vi "Camera.Piezo.vi"() -> ()   [LabVIEW 2015]
uses:
  Camera Properties.ctl
  CameraState.ctl
  CameraControlTypeDef.ctl
  Stack_State.ctl
  Stack Track.ctl
  <vilib>/vision/NI_Vision_Development_Module.lvlib
panel:
  in  "Tab Control":enum32{"Camera Settings", "Recording"}(tab)
  in  "Camera Mode":T1(ring)
  in  "Slit Width /px":dbl
  out "error IO":errorcluster
  in  "V Height":dbl=2048.0 min=4.0 max=2048.0 step=4.0
  in  "V Offset":dbl min=0.0 max=0.0 step=4.0
  in  "H Offset":dbl min=0.0 max=0.0 step=4.0
  in  "H Width":dbl min=4.0 max=2048.0 step=4.0
  in  "Exposure /ms":dbl min=0.0010036691729323308 max=10.000004210526315 step=1e-08
  in  "Trigger Source":dbl(ring)=2.0 items=["Internal"=1.0, "External"=2.0]
  in  "Readout Direction":dbl(ring)=2.0 items=["Forward"=1.0, "Backward"=2.0]
  in  "Scanning Mode":dbl(ring)=12.0 items=["Full Frame"=1.0, "Slit Scanning"=12.0]
  in  "Advanced DCAM Controls":i32(listbox) caption="Multicolumn Listbox"
  in  "Properties":T2=4211904 items=["SENSOR MODE"=4212128, "CCD MODE"=4212384, "READOUT MODE"=4211872, "ACTIVE VIEW INDEX"=4343136, "BITS PER CHANNEL"=4342976, "IMAGE PIXEL TYPE"=4343296, "BINNING"=4215968, "EXPOSURE TIME"=2049184, "CONTRAST GAIN"=3163312, "CONTRAST OFFSET"=3163328, "LIGHT MODE"=2114720, "SENSITIVITY"=2114992, "PHOTON IMAGING MODE"=2115200, "HIGH DYNAMIC RANGE MODE"=3163360, "WHITE BALANCE"=3163568, "TEMPERATURE"=2115232, "TEMPERATURE TARGET"=2115264, "SENSOR COOLER FAN"=2115296, "LINEBUNDLE HEIGHT"=4212192, "MECHANICAL SHUTTER"=2115488, "BACK FOCUS POSITION"=8422304, "TRIGGER CONNECTOR"=1066432, "TRIGGER SOURCE"=1066144, "OUTPUT TRIGGER SOURCE"=1852576, "TRIGGER GLOBAL EXPOSURE"=2049680, "FIRST TRIGGER BEHAVIOR"=2049696, "CHANNEL SYNC"=1852352, "READOUT DIRECTION"=4211904, "PRE HSYNC COUNT"=1852704, "INTERNAL LINE SPEED"=4191408, "INTERNAL LINE INVERVAL"=4191424]
  out "Image":T3(plugin-control)
  out "Histogram":T4(graph)
  in  "stop":bool
  in  "Calibration":bool
  in  "MultiD Scan":bool
  in  "Stage Controller":bool
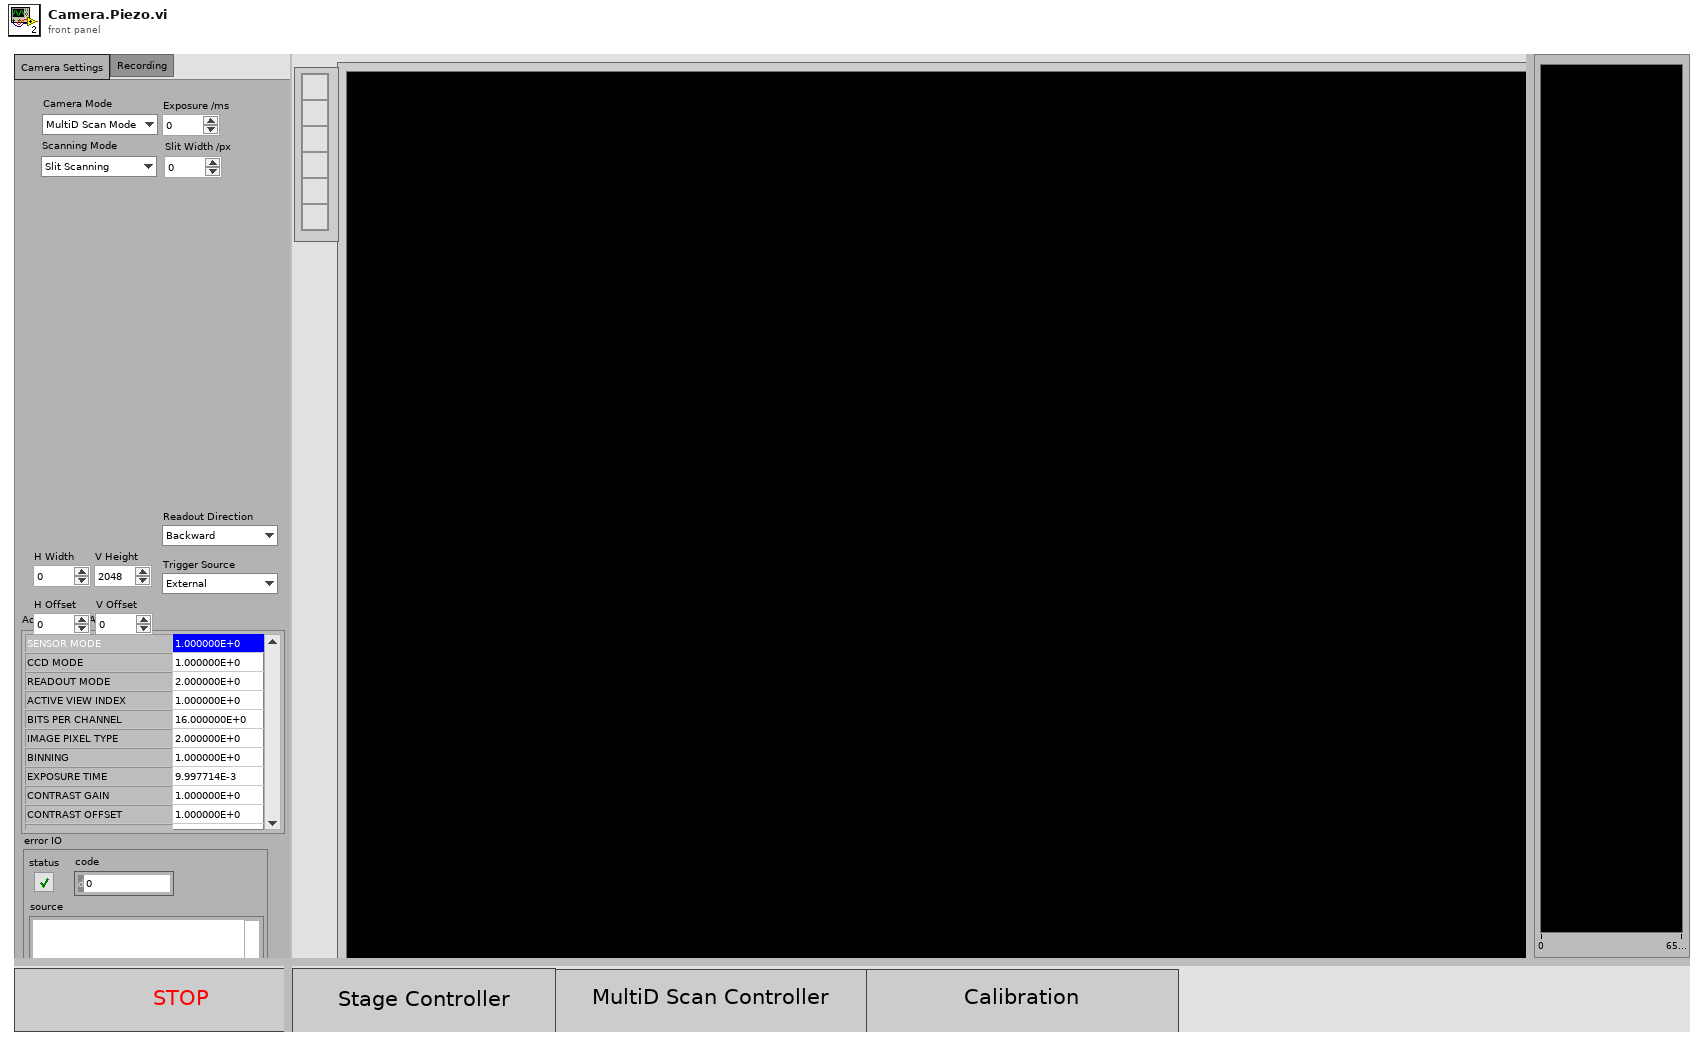
[diagram p1: front panel]
types:
  T1 = enum16{"MultiD Scan Mode", "2D Scan Mode", "Calibration Mode"}
  T2 = typedef "Camera Properties.ctl" = u32
  T3 = typedef "IMAQ Image.ctl" = refnum<image>
  T4 = cluster{"Starting Value":sgl, "Incremental Value":sgl, "Histogram":u32[]}
  T5 = typedef "CameraControlTypeDef.ctl" = enum16{"IntervalLineInt", "Ram Record", "HardDisk Record", "Disengage Update", "Update", "Idle", "ROI", "Binning", "Scan Mode", "Trigger Mode", "Readout Mode", "Readout Direction", "Preview", "ROIWindow", "Trigger Source"}
  T6 = cluster{"height":u32, "width":u32, "datatype":u32}
  T7 = typedef "Stack_State.ctl" = cluster{"State":T8, "Stack Number":i32, "Image":u16[][], "Stacks":i32}
  T8 = typedef "Stack Track.ctl" = enum16{"Idle", "Display", "Start Sequence", "Read Disk", "STOP", "Collecting", "End"}
  T9 = typedef "CameraState.ctl" = enum16{"init", "active", "deinit"}
  T10 = typedef "Image Type" = u32
  T11 = cluster{"Value":i32, "Minimum":i32, "Maximum":i32, "Increment":i32}
  T12 = cluster{"Minimum":i32, "Maximum":i32, "Increment":i32}
  T13 = cluster{"Enum":T5, dbl, "timeout in ms (-1)":u32}
  T14 = cluster{"State":T8, "Timeout":i32, "Data 16":u16[][], "Timeout":i32}
  T15 = cluster{"Enum":T5, "Trigger Source":dbl, "timeout in ms (-1)":i32}
  T16 = cluster{"Enum":T5, "Exposure /ms":dbl, "Parameter":u32}
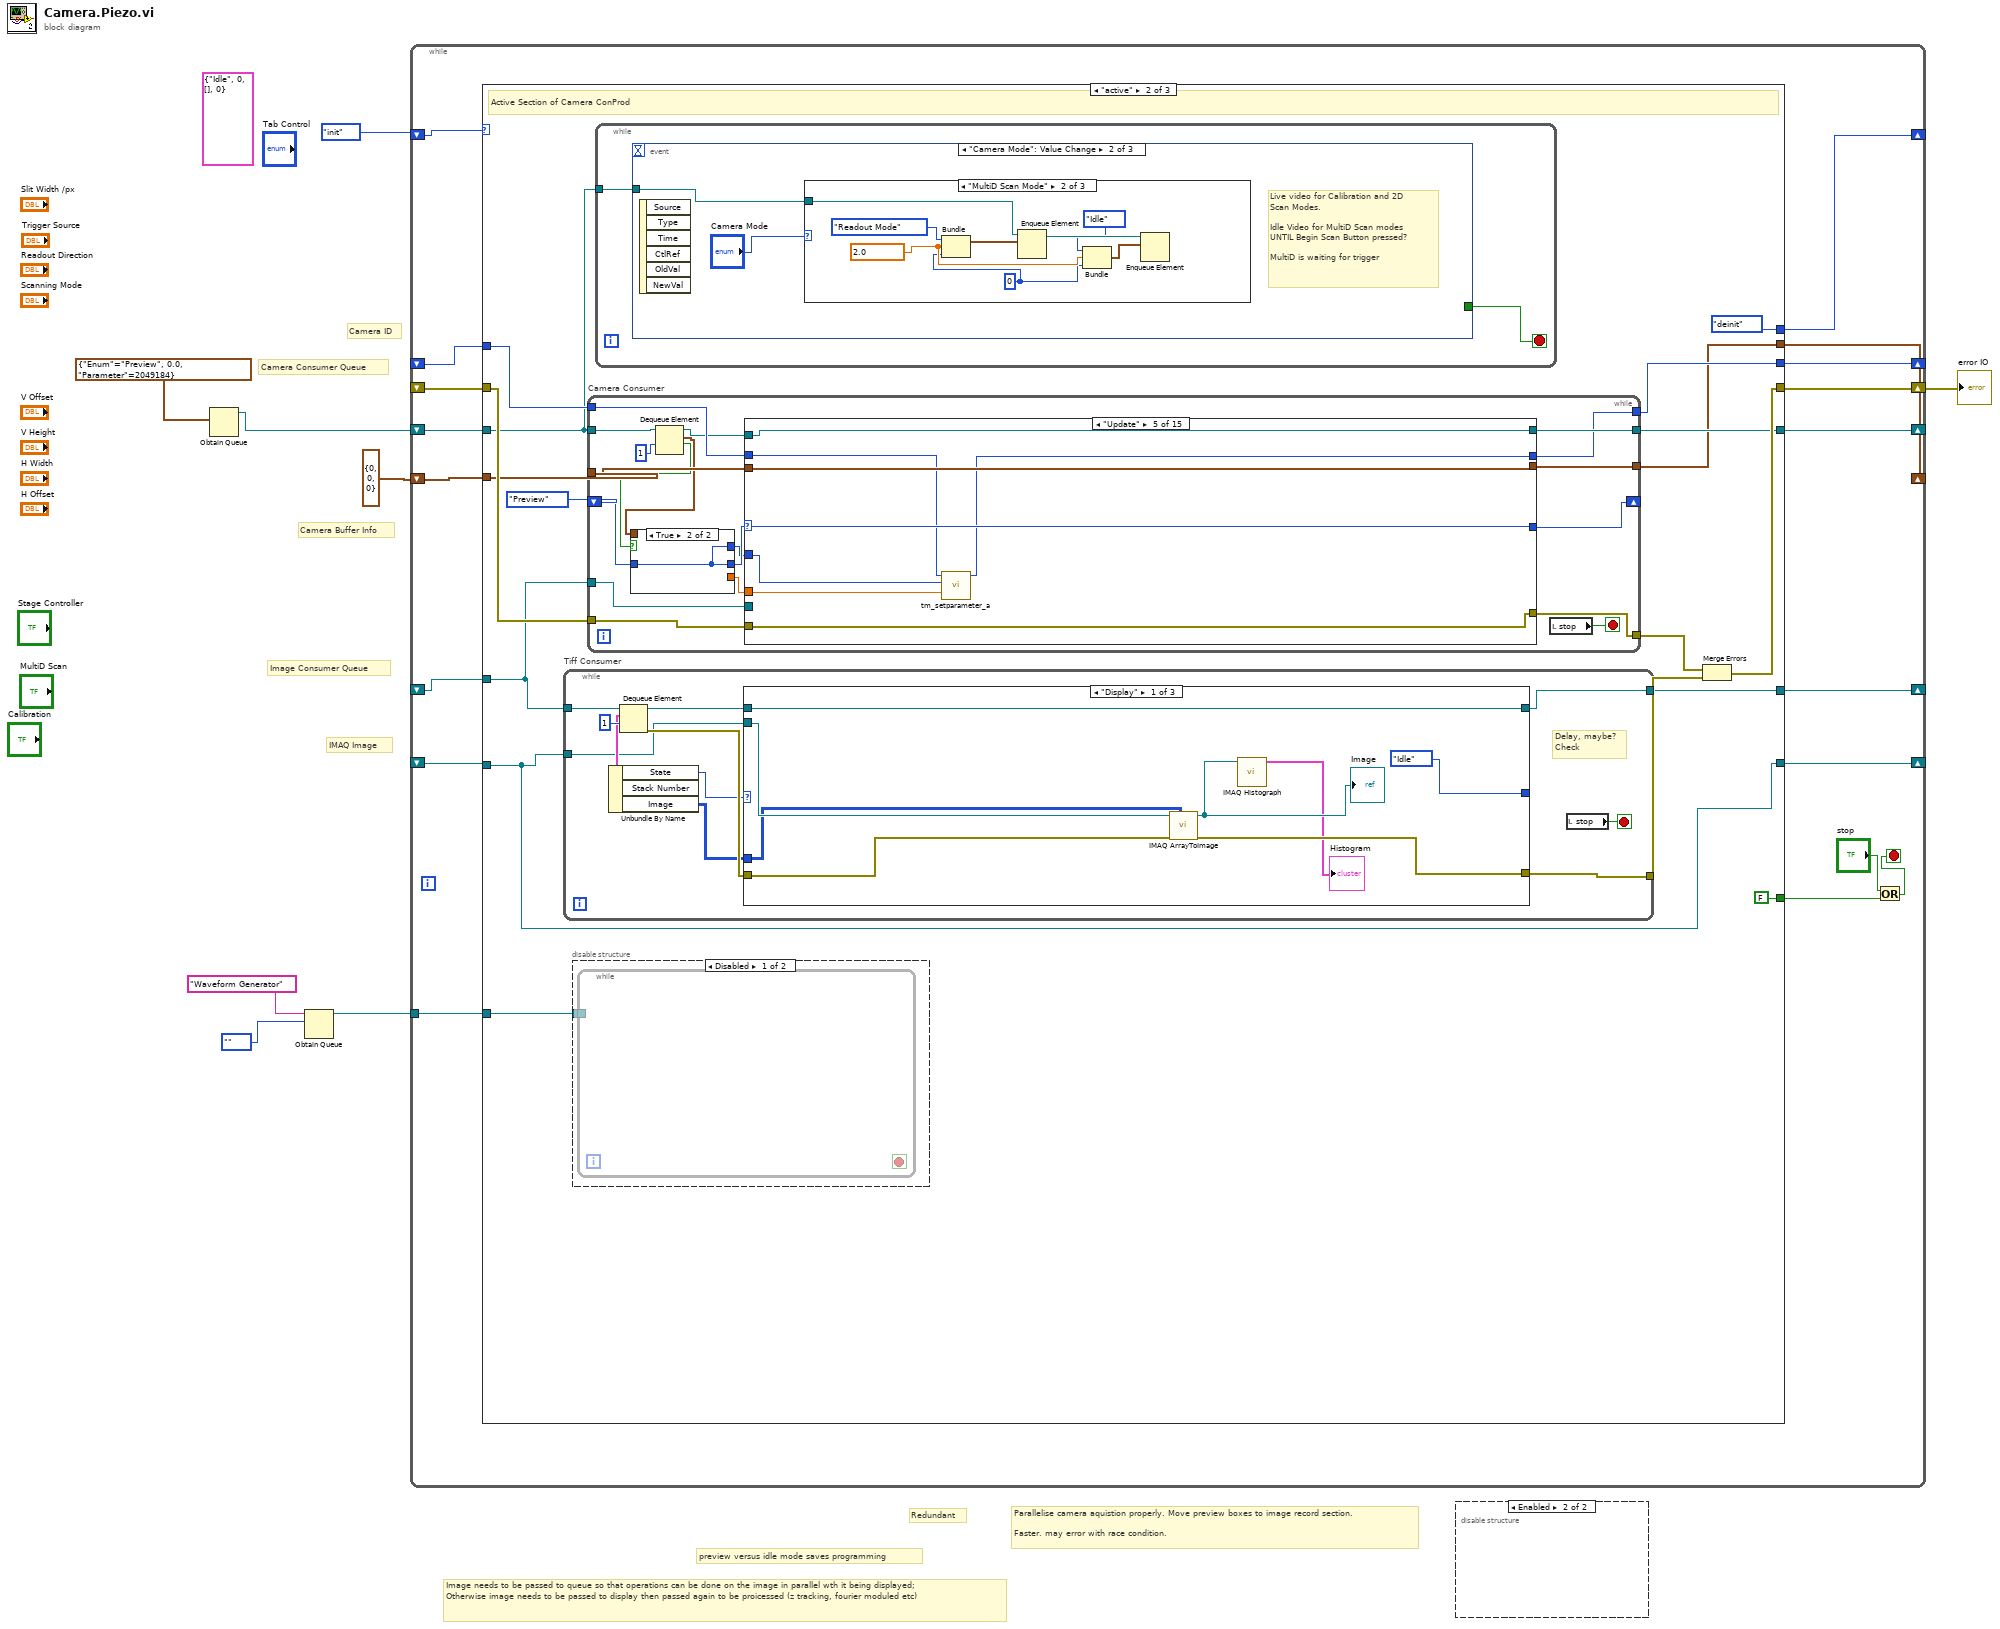
[diagram p0: block diagram]
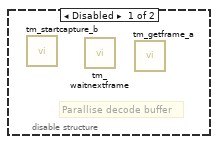
[diagram p2: hidden frame]
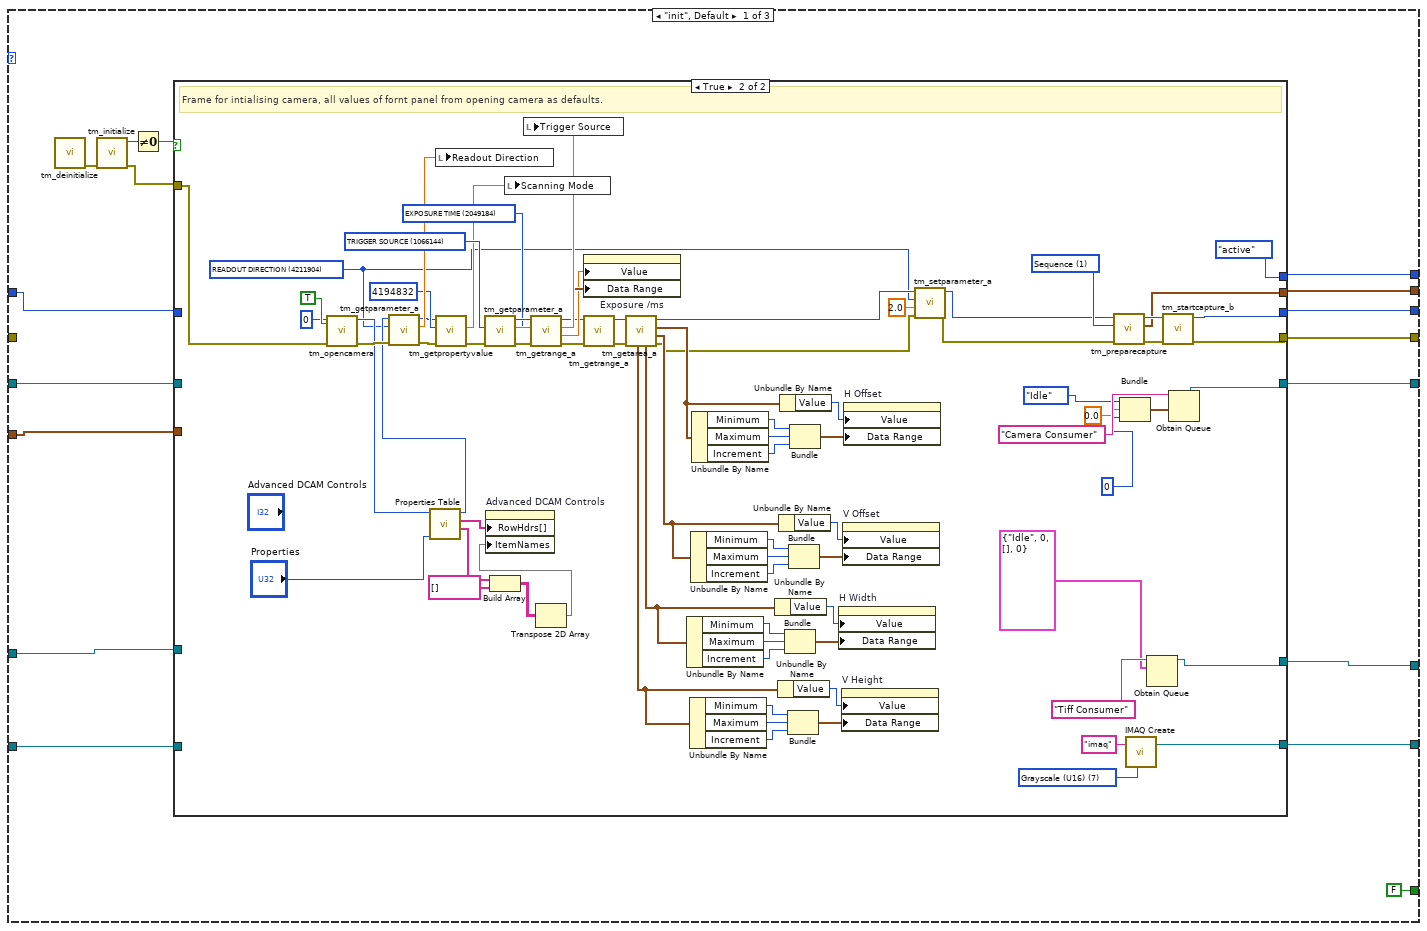
[diagram p3: hidden frame]
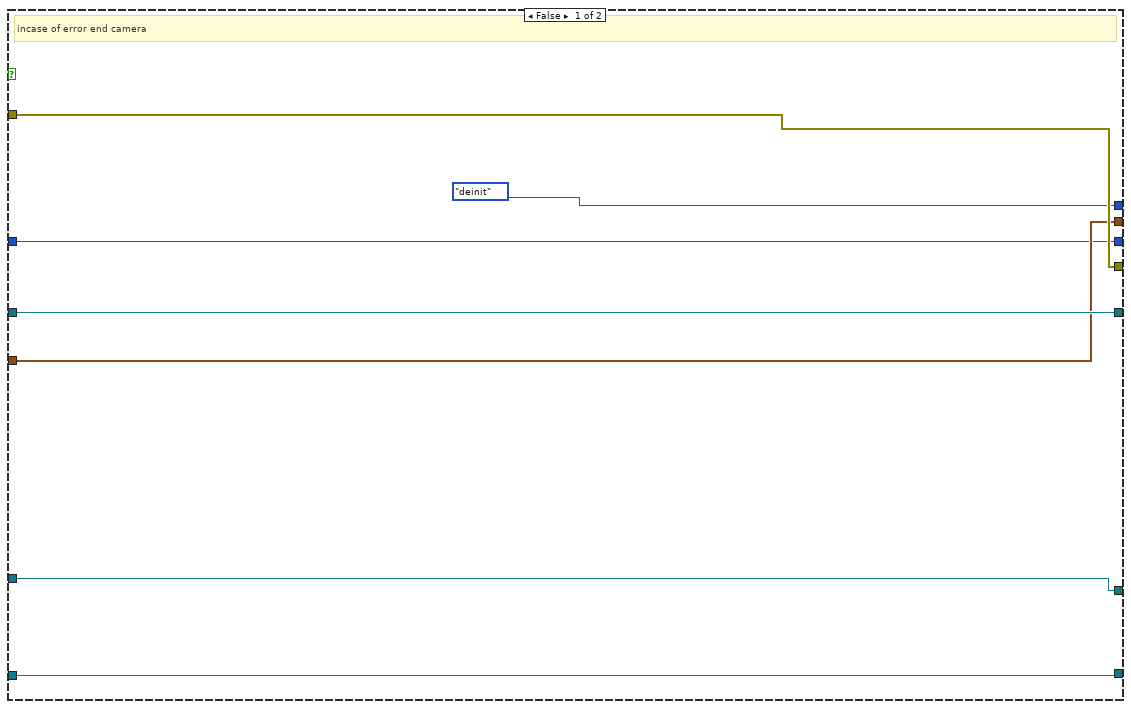
[diagram p4: hidden frame]
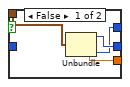
[diagram p8: hidden frame]
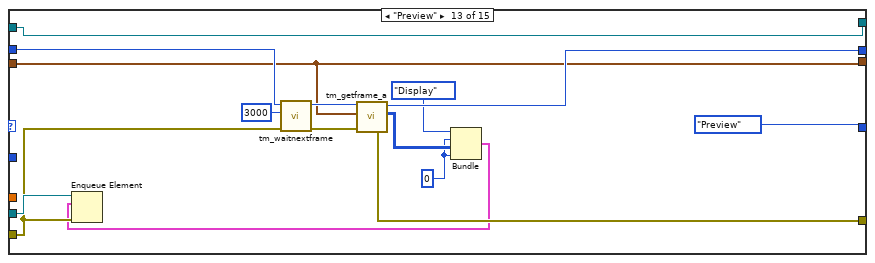
[diagram p20: hidden frame]
diagram:
  (unwired) T7 {"State"=enum."Idle", "Stack Number"=0, "Image"=[], "Stacks"=0} ("input cluster")
  # "IMAQ Image"
  # "Camera Buffer Info"
  # "Image needs to be passed to queue so that operations can be done on the image in parallel wth it being displayed;\nOtherwise image needs to be passed to display then passed again to be proicessed (z tracking, fourier moduled etc)"
  # "preview versus idle mode saves programming"
  # "Parallelise camera aquistion properly. Move preview boxes to image record section.\n\nFaster. may error with race condition."
  # "Redundant"
  # "Image Consumer Queue"
  # "Camera Consumer Queue"
  # "Camera ID"
  n1 = Obtain Queue(element data type=cluster{"Enum":T5, dbl, "Parameter":u32} {"Enum"=enum."Preview", 0.0, "Parameter"=2049184}) -> (queue out=w3:refnum<queue>)  [unwired: 4 in, 2 out]
  n2 = Obtain Queue(name (unnamed)="Waveform Generator", element data type=enum16{""}."") -> (queue out=w2:refnum<queue>)  [unwired: 3 in, 2 out]
  n3 = while {
    shift-right: [w26] -> _
    shift-left: CameraState."init" -> [w25]
    shift-right: [w24] -> _
    shift-left: _ -> [w23]
    shift-right: [w22] -> w7
    shift-left: _ -> [w21]
    shift-right: [w19] -> _
    shift-left: _ -> [w18]
    shift-right: [w20] -> _
    shift-left: w3 -> [w17]
    shift-right: [w13] -> _
    shift-left: T6 {"height"=0, "width"=0, "datatype"=0} ("Buffer Info") -> [w12]
    shift-right: [w11] -> _
    shift-left: _ -> [w10]
    tunnel: w2 -> [w9]
    stop <- w15 stop-if-true
    n4 = case shown="\"active\"" w25 {
      tunnel: [w39 CameraState."deinit" CameraState."init"] -> w26
      tunnel: [w38 w144 w324] -> w24
      tunnel: w23 -> [w29 w145 w324]
      tunnel: [w37 w143 w327] -> w22
      tunnel: w21 -> [_ w137 w328]
      tunnel: [w36 w140 w321] -> w20
      tunnel: [w35 w139 w322] -> w19
      tunnel: w18 -> [w33 w132 w322]
      tunnel: w17 -> [w34 w130 w321]
      tunnel: [FALSE ("stop") FALSE ("stop") TRUE ("stop")] -> w14
      tunnel: [w31 w135 w319] -> w13
      tunnel: w12 -> [w30 w134 w319]
      tunnel: w10 -> [w27 w131 w318]
      tunnel: [w28 w131 w318] -> w11
      tunnel: w9 -> [_ w129 _]
      frame "init", Default {
        n5 = call "tm_deinitialize.vi"() -> ("error out"=w43:errorcluster)  [unwired: 11 in]
        n6 = call "tm_initialize.vi"("error in (no error)"=w43) -> ("error out"=w40:errorcluster, "Number Of Cameras"=w42:u32)  [unwired: 7 in, 2 out]
        n7 = Not Equal To 0?(x=w42) -> (x != 0?=w41:bool)
        n8 = case shown="True" w41 {
          tunnel: w40 -> [w50 w122]
          tunnel: [CameraState."deinit" CameraState."active"] -> w39
          tunnel: [w50 w105] -> w37
          tunnel: [w45 w103] -> w38
          tunnel: [w48 w77] -> w36
          tunnel: [w47 w75] -> w35
          tunnel: w34 -> [w48 _]
          tunnel: w33 -> [w47 _]
          tunnel: [w46 w65] -> w31
          tunnel: w30 -> [w46 _]
          tunnel: w29 -> [w45 _]
          tunnel: [w44 w62] -> w28
          tunnel: w27 -> [w44 _]
          frame False {
            # "incase of error end camera"
          }
          frame True {
            w64 = T10 7 items=["Grayscale (U8)", "Grayscale (I16)", "Grayscale (SGL)", "Complex (CSG)", "RGB (U32)", "HSL (U32)", "RGB (U64)", "Grayscale (U16)"] ("Image Type")
            w107 = 1 items=["Snap", "Sequence"] ("Capture mode")
            w119 = u32 2049184 items=["SENSOR MODE"=4212128, "CCD MODE"=4212384, "READOUT MODE"=4211872, "ACTIVE VIEW INDEX"=4343136, "BITS PER CHANNEL"=4342976, "IMAGE PIXEL TYPE"=4343296, "BINNING"=4215968, "EXPOSURE TIME"=2049184, "CONTRAST GAIN"=3163312, "CONTRAST OFFSET"=3163328, "LIGHT MODE"=2114720, "SENSITIVITY"=2114992, "PHOTON IMAGING MODE"=2115200, "HIGH DYNAMIC RANGE MODE"=3163360, "WHITE BALANCE"=3163568, "TEMPERATURE"=2115232, "TEMPERATURE TARGET"=2115264, "SENSOR COOLER FAN"=2115296, "LINEBUNDLE HEIGHT"=4212192, "MECHANICAL SHUTTER"=2115488, "BACK FOCUS POSITION"=8422304, "TRIGGER CONNECTOR"=1066432, "TRIGGER SOURCE"=1066144, "OUTPUT TRIGGER SOURCE"=1852576, "TRIGGER GLOBAL EXPOSURE"=2049680, "FIRST TRIGGER BEHAVIOR"=2049696, "CHANNEL SYNC"=1852352, "READOUT DIRECTION"=4211904, "PRE HSYNC COUNT"=1852704, "INTERNAL LINE SPEED"=4191408, "INTERNAL LINE INVERVAL"=4191424] ("Parameter")
            w57 = T2 4211904 items=["SENSOR MODE"=4212128, "CCD MODE"=4212384, "READOUT MODE"=4211872, "ACTIVE VIEW INDEX"=4343136, "BITS PER CHANNEL"=4342976, "IMAGE PIXEL TYPE"=4343296, "BINNING"=4215968, "EXPOSURE TIME"=2049184, "CONTRAST GAIN"=3163312, "CONTRAST OFFSET"=3163328, "LIGHT MODE"=2114720, "SENSITIVITY"=2114992, "PHOTON IMAGING MODE"=2115200, "HIGH DYNAMIC RANGE MODE"=3163360, "WHITE BALANCE"=3163568, "TEMPERATURE"=2115232, "TEMPERATURE TARGET"=2115264, "SENSOR COOLER FAN"=2115296, "LINEBUNDLE HEIGHT"=4212192, "MECHANICAL SHUTTER"=2115488, "BACK FOCUS POSITION"=8422304, "TRIGGER CONNECTOR"=1066432, "TRIGGER SOURCE"=1066144, "OUTPUT TRIGGER SOURCE"=1852576, "TRIGGER GLOBAL EXPOSURE"=2049680, "FIRST TRIGGER BEHAVIOR"=2049696, "CHANNEL SYNC"=1852352, "READOUT DIRECTION"=4211904, "PRE HSYNC COUNT"=1852704, "INTERNAL LINE SPEED"=4191408, "INTERNAL LINE INVERVAL"=4191424] ("Parameter")
            w125 = u32 1066144 items=["SENSOR MODE"=4212128, "CCD MODE"=4212384, "READOUT MODE"=4211872, "ACTIVE VIEW INDEX"=4343136, "BITS PER CHANNEL"=4342976, "IMAGE PIXEL TYPE"=4343296, "BINNING"=4215968, "EXPOSURE TIME"=2049184, "CONTRAST GAIN"=3163312, "CONTRAST OFFSET"=3163328, "LIGHT MODE"=2114720, "SENSITIVITY"=2114992, "PHOTON IMAGING MODE"=2115200, "HIGH DYNAMIC RANGE MODE"=3163360, "WHITE BALANCE"=3163568, "TEMPERATURE"=2115232, "TEMPERATURE TARGET"=2115264, "SENSOR COOLER FAN"=2115296, "LINEBUNDLE HEIGHT"=4212192, "MECHANICAL SHUTTER"=2115488, "BACK FOCUS POSITION"=8422304, "TRIGGER CONNECTOR"=1066432, "TRIGGER SOURCE"=1066144, "OUTPUT TRIGGER SOURCE"=1852576, "TRIGGER GLOBAL EXPOSURE"=2049680, "FIRST TRIGGER BEHAVIOR"=2049696, "CHANNEL SYNC"=1852352, "READOUT DIRECTION"=4211904, "PRE HSYNC COUNT"=1852704, "INTERNAL LINE SPEED"=4191408, "INTERNAL LINE INVERVAL"=4191424] ("Parameter")
            # "Frame for intialising camera, all values of fornt panel from opening camera as defaults."
            n9 = call "tm_opencamera.vi"("Force Open"=TRUE, "error in (no error)"=w122, "Camera Index"=u32 0) -> ("error out"=w126:errorcluster, "Handle out"=w73:u32)  [unwired: 6 in, 1 out]
            n10 = call "Properties Table.vi"("Properties"="Properties", "Handle In"=w73) -> ("Value Stirngs Out"=w70:string[], "Row Headers"=w71:string[], "Handle Out"=w72:u32)  [unwired: 3 in, 1 out]
            n11 = call "tm_getparameter_a.vi"("error in (no error)"=w126, "Parameter"=w57, "Handle in"=w72) -> ("error out"=w108:errorcluster, "Value out"=w123:dbl, "Handle out"=w111:u32)  [unwired: 6 in]
            n12 = local write "Readout Direction"(w123) -> ()
            n13 = call "tm_getpropertyvalue.vi"("error in (no error)"=w108, "Property ID"=u32 4194832, "Handle in"=w111) -> ("error out"=w109:errorcluster, "Value in"=w110:sgl)  [unwired: 6 in, 1 out]
            n14 = call "tm_getparameter_a.vi"("error in (no error)"=w109, "Parameter"=w125) -> ("error out"=w120:errorcluster, "Value out"=w124:dbl, "Handle out"=w121:u32)  [unwired: 7 in]
            n15 = Build Array(w70, string[] [] ("element")) -> (w68:string[][])
            n16 = local write "Scanning Mode"(w110) -> ()
            n17 = local write "Trigger Source"(w124) -> ()
            n18 = call "tm_getrange_a.vi"("error in (no error)"=w120, "Parameter"=w119, "Handle in"=w121) -> ("error out"=w115:errorcluster, "default"=w117:dbl, "Range"=w118:cluster{"min":dbl, "max":dbl, "step":dbl}, "Handle out"=w116:u32)  [unwired: 2 in, 3 out]
            n19 = Transpose 2D Array(2D array=w68) -> (transposed array=w67:string[][])
            n20 = property on="Advanced DCAM Controls" class="MCListbox (strict)"("RowHdrs[]"=w71, "ItemNames"=w67) -> ()  [unwired: 2 in, 2 out]
            n21 = property on="Exposure /ms" class="DigNum (strict)"("Value"=w117, "Data Range"=w118) -> ()  [unwired: 2 in, 2 out]
            n22 = call "tm_getrange_a.vi"("error in (no error)"=w115, "Handle in"=w116) -> ("error out"=w114:errorcluster, "Handle out"=w113:u32)  [unwired: 3 in, 5 out]
            n23 = call "tm_getarea_a.vi"("error in (no error)"=w114, "Handle in"=w113) -> ("error out"=w59:errorcluster, "V Offset"=w79:T11, "H Offset"=w102:T11, "Handle out"=w61:u32, "H Width"=w80:T11, "V Width"=w81:T11)  [unwired: 4 in]
            n24 = Unbundle By Name(w80) -> ("Minimum"=w91:i32, "Maximum"=w90:i32, "Increment"=w89:i32)
            n25 = Unbundle By Name(w81) -> ("Minimum"=w82:i32, "Maximum"=w83:i32, "Increment"=w84:i32)
            n26 = Unbundle By Name(w79) -> ("Minimum"=w92:i32, "Maximum"=w93:i32, "Increment"=w94:i32)
            n27 = Unbundle By Name(w102) -> ("Minimum"=w101:i32, "Maximum"=w100:i32, "Increment"=w99:i32)
            n28 = Unbundle By Name(w80) -> ("Value"=w87:i32)
            n29 = Unbundle By Name(w81) -> ("Value"=w86:i32)
            n30 = Unbundle By Name(w79) -> ("Value"=w96:i32)
            n31 = Unbundle By Name(w102) -> ("Value"=w97:i32)
            n32 = Bundle("Minimum"=w91, "Maximum"=w90, "Increment"=w89) -> (w88:T12)  [unwired: 1 in]
            n33 = Bundle("Minimum"=w82, "Maximum"=w83, "Increment"=w84) -> (w85:T12)  [unwired: 1 in]
            n34 = Bundle("Minimum"=w92, "Maximum"=w93, "Increment"=w94) -> (w95:T12)  [unwired: 1 in]
            n35 = Bundle("Minimum"=w101, "Maximum"=w100, "Increment"=w99) -> (w98:T12)  [unwired: 1 in]
            n36 = property on="H Width" class="DigNum (strict)"("Value"=w87, "Data Range"=w88) -> ()  [unwired: 2 in, 2 out]
            n37 = property on="V Height" class="DigNum (strict)"("Value"=w86, "Data Range"=w85) -> ()  [unwired: 2 in, 2 out]
            n38 = property on="V Offset" class="DigNum (strict)"("Value"=w96, "Data Range"=w95) -> ()  [unwired: 2 in, 2 out]
            n39 = property on="H Offset" class="DigNum (strict)"("Value"=w97, "Data Range"=w98) -> ()  [unwired: 2 in, 2 out]
            n40 = call "tm_setparameter_a.vi"("error in (no error)"=w59, "Value in"=2.0, "Parameter"=w57, "Handle in"=w61) -> ("error out"=w58:errorcluster, "Handle out"=w60:u32)  [unwired: 6 in]
            n41 = call "tm_preparecapture.vi"("error in (no error)"=w58, "Capture mode"=w107, "Handle in"=w60) -> ("error out"=w106:errorcluster, "Buffer Info"=w65:T6, "Handle out"=w104:u32)  [unwired: 5 in, 1 out]
            n42 = Bundle("Enum"=CameraControlTypeDef."Idle", 0.0, "timeout in ms (-1)"=u32 0) -> (w53:T13)  [unwired: 1 in]
            n43 = call "IMAQ Create"("Image Name"="imaq", "Image Type"=w64) -> ("New Image"=w62:T3)  [unwired: 3 in, 1 out]
            n44 = Obtain Queue(name (unnamed)="Tiff Consumer", element data type=T7 {"State"=enum."Idle", "Stack Number"=0, "Image"=[], "Stacks"=0} ("input cluster")) -> (queue out=w75:refnum<queue>)  [unwired: 3 in, 2 out]
            n45 = call "tm_startcapture_b.vi"("error in (no error)"=w106, "Handle in"=w104) -> ("error out"=w105:errorcluster, "Handle out"=w103:u32)  [unwired: 8 in]
            n46 = Obtain Queue(name (unnamed)="Camera Consumer", element data type=w53) -> (queue out=w77:refnum<queue>)  [unwired: 3 in, 2 out]
          }
        }
      }
      frame "active" {
        # "Active Section of Camera ConProd"
        n47 = while "Tiff Consumer" {
          tunnel: [w150] -> w142
          tunnel: [w153] -> w139
          tunnel: w132 -> [w155]
          tunnel: w131 -> [w147]
          stop <- w157 stop-if-true
          # "Delay, maybe?\nCheck"
          n48 = Dequeue Element(queue=w155, timeout in ms (-1)=1) -> (queue out=w152:refnum<queue>, element=w154:T7, error out=w151:errorcluster)  [unwired: 1 in, 1 out]
          n49 = Unbundle By Name(w154) -> ("State"=w148:T8, "Image"=w149:u16[][])  [unwired: 1 out]
          n50 = case shown="\"Display\"" w148 {
            selector: w148 -> [_ w168 w169]
            tunnel: [w165 w167 w170] -> w153
            tunnel: w152 -> [w165 w167 w170]
            tunnel: [Stack_Track."Idle" ("State") w168 w169] -> _
            tunnel: w149 -> [w160 _ _]
            tunnel: w147 -> [w164 _ _]
            tunnel: w151 -> [w163 w166 w171]
            tunnel: [w162 w166 w171] -> w150
            frame "Display" {
              n51 = call "IMAQ ArrayToImage"("Image Pixels (U16)"=w160, "error in (no error)"=w163, "Image"=w164) -> ("error out"=w162:errorcluster, "Image Out"=w159:T3)  [unwired: 7 in]
              "Image" <- w159
              n52 = call "IMAQ Histograph"("Image"=w159) -> ("Histogram Graph"=→"Histogram":T4)  [unwired: 7 in, 3 out]
            }
            frame "Idle", Default {
            }
            frame "Start Sequence" {
            }
          }
          n53 = local read "stop"() -> (w157:bool)
        }
        n54 = disable-structure shown="Disabled" {
          disable-tunnel: w129 -> [w146 _]
          frame Disabled {
            n55 = while {
              tunnel: w146 -> [_]
              stop <- _ stop-if-true
            }
          }
          frame Enabled {
          }
        }
        n56 = while "Camera Consumer" {
          tunnel: w137 -> [w188]
          tunnel: w145 -> [w185]
          tunnel: [w184] -> w144
          tunnel: [w187] -> w141
          tunnel: w130 -> [w180]
          tunnel: [w189] -> w140
          shift-right: [w186] -> _
          shift-left: CameraControlTypeDef."Preview" ("Enum") -> [w176]
          tunnel: [w183] -> w135
          tunnel: w134 -> [w182]
          tunnel: w132 -> [w175]
          stop <- w190 stop-if-true
          n57 = Dequeue Element(queue=w180, timeout in ms (-1)=1) -> (queue out=w179:refnum<queue>, element=w174:cluster{"Enum":T5, dbl, "Parameter":u32}, timed out?=w178:bool)  [unwired: 1 in, 1 out]
          n58 = case shown="True" w178 {
            tunnel: [w193 w195] -> w177
            tunnel: w176 -> [_ w195]
            tunnel: w174 -> [w194 _]
            tunnel: [w192 _] -> w173
            tunnel: [w191 w195] -> w172
            frame False {
              n59 = Unbundle(w194) -> ("Enum"=w193:T5, w192:dbl, "Parameter"=w191:u32)
            }
            frame True {
            }
          }
          n60 = case shown="\"Update\"" w177 {
            selector: w177 -> [w199 w204 w209 w214 w222 w227 w232 w237 w242 w247 w252 w257 _ w276 _]
            tunnel: w179 -> [w198 w205 w210 w215 w223 w228 w233 w238 w243 w248 w253 w258 w273 w278 w283]
            tunnel: [w198 w205 w210 w215 w223 w228 w233 w238 w243 w248 w253 w258 w273 w278 w283] -> w189
            tunnel: w188 -> [w200 w203 w208 w213 w221 w226 w231 w236 w241 w246 w251 w256 w263 w275 w281]
            tunnel: [w200 w203 w208 w213 w221 w226 w231 w236 w241 w246 w251 w256 w267 w275 w281] -> w187
            tunnel: [w199 w204 w209 w214 w222 w227 w232 w237 w242 w247 w252 w257 CameraControlTypeDef."Preview" ("Enum") w276 CameraControlTypeDef."Preview" ("Enum")] -> w186
            tunnel: w185 -> [w197 w202 w207 w212 w219 w225 w230 w235 w240 w245 w250 w255 w271 w277 w282]
            tunnel: [w197 w202 w207 w212 w218 w225 w230 w235 w240 w245 w250 w255 w269 w277 w282] -> w184
            tunnel: [w196 w201 w206 w211 w220 w224 w229 w234 w239 w244 w249 w254 w265 w274 w280] -> w183
            tunnel: w182 -> [w196 w201 w206 w211 w220 w224 w229 w234 w239 w244 w249 w254 w265 w274 w280]
            tunnel: w175 -> [_ _ _ _ _ _ _ _ _ _ _ _ w264 _ _]
            tunnel: w173 -> [_ _ _ _ w216 _ _ _ _ _ _ _ _ _ _]
            tunnel: w172 -> [_ _ _ _ w217 _ _ _ _ _ _ _ _ _ _]
            frame "IntervalLineInt" {
            }
            frame "Ram Record" {
            }
            frame "HardDisk Record" {
            }
            frame "Disengage Update" {
            }
            frame "Update" {
              n61 = call "tm_setparameter_a.vi"("Value in"=w216, "Parameter"=w217, "Handle in"=w219) -> ("Handle out"=w218:u32)  [unwired: 7 in, 1 out]
            }
            frame "Idle", Default {
            }
            frame "ROI" {
            }
            frame "Binning" {
            }
            frame "Scan Mode" {
            }
            frame "Trigger Mode" {
            }
            frame "Readout Mode" {
            }
            frame "Readout Direction" {
            }
            frame "Preview" {
              w260 = 0 ("Timeout")
              n62 = call "tm_waitnextframe.vi"("error in (no error)"=w263, "Timeout"=3000, "Handle in"=w271) -> ("error out"=w268:errorcluster, "Handle out"=w270:u32)  [unwired: 5 in, 2 out]
              n63 = call "tm_getframe_a.vi"("error in (no error)"=w268, "Buffer Info"=w265, "Handle in"=w270) -> ("error out"=w267:errorcluster, "Data 16"=w261:u16[][], "Handle out"=w269:u32)  [unwired: 4 in, 2 out]
              n64 = Bundle("State"=Stack_Track."Display", "Timeout"=w260, "Data 16"=w261, "Timeout"=w260) -> (w259:T14)  [unwired: 1 in]
              n65 = Enqueue Element(queue=w264, element=w259, error in (no error)=w263) -> ()  [unwired: 1 in, 3 out]
            }
            frame "ROIWindow" {
            }
            frame "Trigger Source" {
              n66 = call "tm_unpreparecapture.vi"() -> ()  [unwired: 10 in, 2 out]
              n67 = call "tm_setparameter_a.vi"() -> ()  [unwired: 10 in, 2 out]
              n68 = call "tm_preparecapture.vi"() -> ()  [unwired: 8 in, 4 out]
            }
          }
          n69 = local read "stop"() -> (w190:bool)
        }
        n70 = while {
          tunnel: w130 -> [w284]
          stop <- w285 stop-if-true
          n71 = event shown="[1] \"Camera Mode\": Value Change" {
            selector: _ -> [_ _ _]
            dyn-events: _ -> [_ _ _]
            timeout: _ -> [_ _ _]
            tunnel: [w286 _ _] -> w285
            tunnel: w284 -> [_ w287 w315]
            event "stop": Value Change {
              n72 = event-data() -> ()  [unwired: 1 in, 6 out]
              n73 = local read "stop"() -> (w286:bool)
            }
            event "Camera Mode": Value Change {
              # "Live video for Calibration and 2D\nScan Modes.\n\nIdle Video for MultiD Scan modes\nUNTIL Begin Scan Button pressed?\n\nMultiD is waiting for trigger"
              n74 = event-data() -> ()  [unwired: 1 in, 6 out]
              n75 = case shown="\"MultiD Scan Mode\"" "Camera Mode" {
                tunnel: w287 -> [w295 w303 w311]
                frame "Calibration Mode" {
                  w289 = 0 ("timeout in ms (-1)")
                  w290 = 1.0 items=["Internal"=1.0, "External"=2.0] ("Trigger Source")
                  n76 = Bundle("Enum"=CameraControlTypeDef."Readout Mode", "Trigger Source"=w290, "timeout in ms (-1)"=w289) -> (w294:T15)  [unwired: 1 in]
                  n77 = Enqueue Element(queue=w295, element=w294) -> (queue out=w292:refnum<queue>)  [unwired: 2 in, 2 out]
                  n78 = Bundle("Enum"=CameraControlTypeDef."Preview", "Trigger Source"=w290, "timeout in ms (-1)"=w289) -> (w293:T15)  [unwired: 1 in]
                  n79 = Enqueue Element(queue=w292, element=w293) -> ()  [unwired: 2 in, 3 out]
                }
                frame "MultiD Scan Mode" {
                  w297 = 0 ("timeout in ms (-1)")
                  w298 = 2.0 items=["Internal"=1.0, "External"=2.0] ("Trigger Source")
                  n80 = Bundle("Enum"=CameraControlTypeDef."Readout Mode", "Trigger Source"=w298, "timeout in ms (-1)"=w297) -> (w302:T15)  [unwired: 1 in]
                  n81 = Enqueue Element(queue=w303, element=w302) -> (queue out=w301:refnum<queue>)  [unwired: 2 in, 2 out]
                  n82 = Bundle("Enum"=CameraControlTypeDef."Idle", "Trigger Source"=w298, "timeout in ms (-1)"=w297) -> (w300:T15)  [unwired: 1 in]
                  n83 = Enqueue Element(queue=w301, element=w300) -> ()  [unwired: 2 in, 3 out]
                }
                frame "2D Scan Mode" {
                  w305 = 0 ("timeout in ms (-1)")
                  w306 = 2.0 items=["Internal"=1.0, "External"=2.0] ("Trigger Source")
                  n84 = Bundle("Enum"=CameraControlTypeDef."Readout Mode", "Trigger Source"=w306, "timeout in ms (-1)"=w305) -> (w310:T15)  [unwired: 1 in]
                  n85 = Enqueue Element(queue=w311, element=w310) -> (queue out=w307:refnum<queue>)  [unwired: 2 in, 2 out]
                  n86 = Bundle("Enum"=CameraControlTypeDef."Preview", "Trigger Source"=w306, "timeout in ms (-1)"=w305) -> (w309:T15)  [unwired: 1 in]
                  n87 = Enqueue Element(queue=w307, element=w309) -> ()  [unwired: 2 in, 3 out]
                }
              }
            }
            event "Exposure /ms": Value Change {
              w313 = u32 2049184 items=["SENSOR MODE"=4212128, "CCD MODE"=4212384, "READOUT MODE"=4211872, "ACTIVE VIEW INDEX"=4343136, "BITS PER CHANNEL"=4342976, "IMAGE PIXEL TYPE"=4343296, "BINNING"=4215968, "EXPOSURE TIME"=2049184, "CONTRAST GAIN"=3163312, "CONTRAST OFFSET"=3163328, "LIGHT MODE"=2114720, "SENSITIVITY"=2114992, "PHOTON IMAGING MODE"=2115200, "HIGH DYNAMIC RANGE MODE"=3163360, "WHITE BALANCE"=3163568, "TEMPERATURE"=2115232, "TEMPERATURE TARGET"=2115264, "SENSOR COOLER FAN"=2115296, "LINEBUNDLE HEIGHT"=4212192, "MECHANICAL SHUTTER"=2115488, "BACK FOCUS POSITION"=8422304, "TRIGGER CONNECTOR"=1066432, "TRIGGER SOURCE"=1066144, "OUTPUT TRIGGER SOURCE"=1852576, "TRIGGER GLOBAL EXPOSURE"=2049680, "FIRST TRIGGER BEHAVIOR"=2049696, "CHANNEL SYNC"=1852352, "READOUT DIRECTION"=4211904, "PRE HSYNC COUNT"=1852704, "INTERNAL LINE SPEED"=4191408, "INTERNAL LINE INTERVAL"=4191424] ("Parameter")
              n88 = event-data() -> ()  [unwired: 1 in, 6 out]
              n89 = Bundle("Enum"=CameraControlTypeDef."Update", "Exposure /ms"="Exposure /ms", "Parameter"=w313) -> (w314:T16)  [unwired: 1 in]
              n90 = Enqueue Element(queue=w315, element=w314) -> ()  [unwired: 2 in, 3 out]
            }
          }
        }
        n91 = Merge Errors(w141, w142) -> (w143:errorcluster)
      }
      frame "deinit" {
        n92 = call "tm_stopcapture.vi"("error in (no error)"=w328, "Handle in"=w324) -> ("error out"=w331:errorcluster, "Handle out"=w330:u32)  [unwired: 8 in]
        n93 = call "tm_unpreparecapture.vi"("error in (no error)"=w331, "Handle in"=w330) -> ("error out"=w332:errorcluster, "Handle out"=w329:u32)  [unwired: 8 in]
        n94 = call "tm_closecamera.vi"("error in (no error)"=w332, "Handle in"=w329) -> ("error out"=w333:errorcluster)  [unwired: 9 in]
        n95 = call "tm_deinitialize.vi"("error in (no error)"=w333) -> ("error out"=w334:errorcluster)  [unwired: 10 in]
        n96 = Release Queue(queue=w322, error in (no error)=w334) -> (error out=w326:errorcluster)  [unwired: 1 in, 2 out]
        n97 = Release Queue(queue=w321, error in (no error)=w334) -> (error out=w325:errorcluster)  [unwired: 1 in, 2 out]
        n98 = Merge Errors(w326, w325) -> (w327:errorcluster)
      }
    }
    n99 = Or(x="stop", y=w14) -> (x .or. y?=w15:bool)
  }
  "error IO" <- w7
  n100 = disable-structure shown="Enabled" {
    frame Disabled {
      # "Parallise decode buffer"
      n101 = call "tm_startcapture_b.vi"() -> ()  [unwired: 10 in, 2 out]
      n102 = call "tm_waitnextframe.vi"() -> ()  [unwired: 8 in, 4 out]
      n103 = call "tm_getframe_a.vi"() -> ()  [unwired: 7 in, 5 out]
    }
    frame Enabled {
    }
  }
